vi "Read Consumer Name.vi"(8 "error in (no error)":errorcluster, 11 "Consumer Name Response Message in":refnum<class "Consumer Name Response Message.lvclass">) -> (0 "error out":errorcluster, 2 "Consumer Name":string, 3 "Consumer Name Response Message out":refnum<class "Consumer Name Response Message.lvclass">)   [LabVIEW 2017, in "Consumer Name Response Message.lvclass"]
uses:
  Consumer Name Response Message.lvclass
  Consumer Name Response Message.lvclass/Consumer Name Response Message.ctl
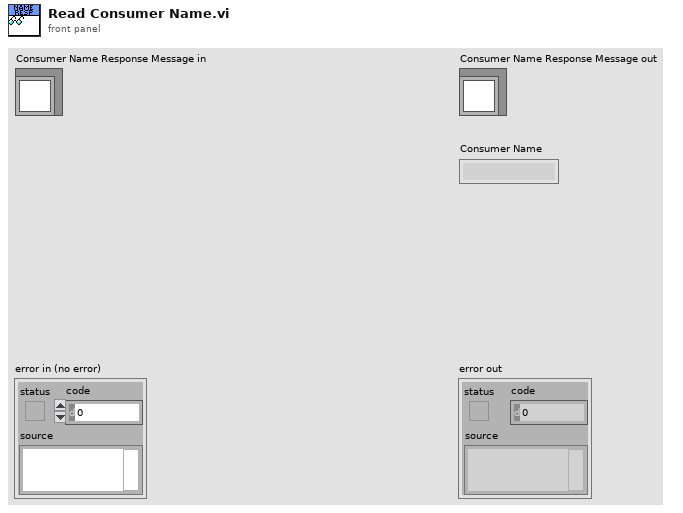
[diagram p1: front panel]
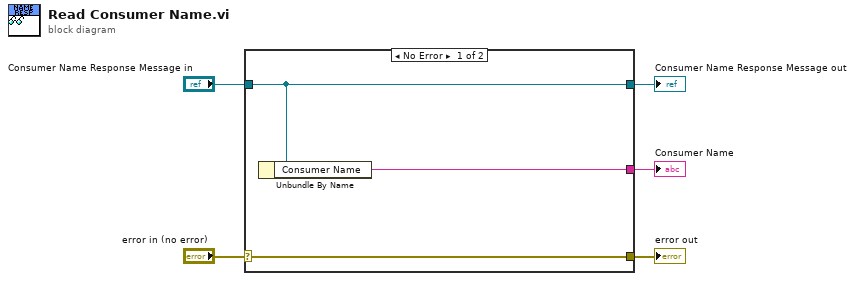
[diagram p0: block diagram]
diagram:
  n1 = case shown="No Error" "error in (no error)" {
    selector: "error in (no error)" -> [w8 w9]
    tunnel: [w8 w9] -> w4
    tunnel: [w7 w10] -> w2
    tunnel: "Consumer Name Response Message in" -> [w7 w10]
    tunnel: [w6 _] -> w1
    frame No Error {
      n2 = Unbundle By Name(w7) -> ("Consumer Name"=w6:string)
    }
    frame Error {
    }
  }
  "error out" <- w4
  "Consumer Name Response Message out" <- w2
  "Consumer Name" <- w1
